vi "Check Text Change.vi"(8 "VKey":T1, 9 "Char":i16=8, 10 "Str Refnum":refnum<vi>, 11 "Data In":string) -> (1 "Text Changed?":bool, 3 "Data Out":string)   [LabVIEW 2011, in "Intellisense Xcontrol.xctl"]
uses:
  Intellisense Xcontrol.xctl
  <vilib>/event_ctls.llb/eventvkey.ctl
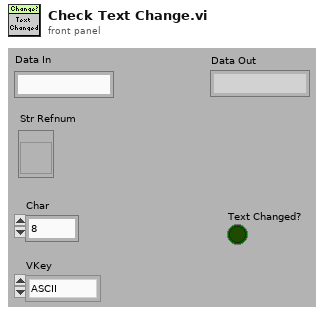
[diagram p1: front panel]
types:
  T1 = typedef "eventvkey.ctl" = enum16{"ASCII", "Enter", "Return", "Shift", "Ctrl", "Alt", "Cmd", "Opt", "Caps", "NumLock", "Clear", "Break", "Up", "Down", "Left", "Right", "Insert", "Delete", "Home", "End", "PageUp", "PageDown", "Escape", "Help", "Pause", "ScrollLock", "F1", "F2", "F3", "F4", "F5", "F6", "F7", "F8", "F9", "F10", "F11", "F12", "F13", "F14", "F15", "F16", "F17", "F18", "F19", "F20", "F21", "F22", "F23", "F24", "Play", "VolumeUp", "VolumeDown", "Mute", "Two Byte Char"}
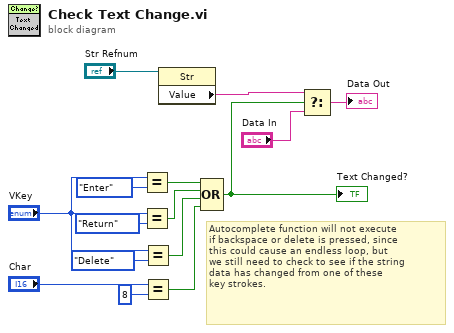
[diagram p0: block diagram]
diagram:
  # "Autocomplete function will not execute\nif backspace or delete is pressed, since\nthis could cause an endless loop, but\nwe still need to check to see if the string\ndata has changed from one of these\nkey strokes."
  n1 = Equal?(x="VKey", y=eventvkey."Enter") -> (x = y?=w9:bool)
  n2 = Equal?(x="VKey", y=eventvkey."Return") -> (x = y?=w8:bool)
  n3 = Equal?(x="VKey", y=eventvkey."Delete") -> (x = y?=w7:bool)
  n4 = Equal?(x="Char", y=i16 8) -> (x = y?=w6:bool)
  n5 = property class="Str"(reference="Str Refnum") -> ("Value"=w4:string)  [unwired: 1 in, 2 out]
  n6 = Compound Arithmetic op=OR(w9, w8, w7, w6) -> (w3:bool)
  "Text Changed?" <- w3
  n7 = Select(t=w4, s=w3, f="Data In") -> (s? t:f=→"Data Out":string)
